vi "Convert dBm to Watt.vi"(4 "dBm":dbl format="%.2f") -> (1 "Watts":dbl format="%.4f")   [LabVIEW 2011]
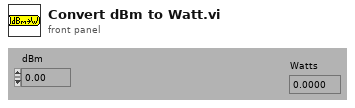
[diagram p1: front panel]
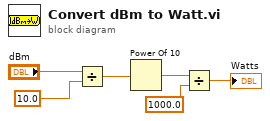
[diagram p0: block diagram]
diagram:
  n1 = Divide(x="dBm", y=10.0) -> (x/y=w5:dbl)
  n2 = Power Of 10(x=w5) -> (10^x=w4:dbl)
  n3 = Divide(x=w4, y=1000.0) -> (x/y=→"Watts":dbl)
